vi "Engine.vi"() -> ()   [LabVIEW 2019]
uses:
  <vilib>/TaskbarProgressAPI/_TypeDefs/Progress State.ctl
  F:/src/Git/machine/CDL0100/TagEngine/LVOPCUA.NET/LVOPC.NETInterface/bin/Release/LVOPC.NETInterface.dll
  LVOPCUA.NET/LVOPC.NETInterface/bin/Release/LVOPC.NETInterface.dll
  <resource>/objmgr/ni.var.rc
  <vilib>/TaskbarProgressAPI/TaskbarProgressAPI.lvlib
panel:
  out "Scada Error":errorcluster
  out "Alarms SVE Size":i32
  out "Alarms Found":i32
  out "Listener ipAddr":string
  out "IP Addresses":string[](array[string])
  out "Basement Anybus OK":bool
  out "Profinet_Slaves_Connected":bool
  out "Profinet_Master_OK":bool
  out "Connected":i32
  out "Sweep Time":dbl(graph)
  out "Variables":i32
  out "Subscriptions":i32
  out "Sessions":i32
  out "Basement Rack Scanner":bool
  out "PLC Sweep Time":dbl
  out "PLC Sweep mode":string
  out "PLC Firmware":string
  out "PLC Date Code":string
  out "PLC Model":string
  out "error IO":errorcluster
  out "Loop Count":i32
  out "PSP Update Tm":dbl format="%#_4g"
  out "Wait Cycles":i32
  in  "stop":bool
  out "error out":errorcluster
  in  "PLC ipAddr":string="192.168.1.15"
  # "ms"
  # "OPC Server"
  # "Max=5"
  # "Max=10"
  # "Max=\n12,500"
  # "ms"
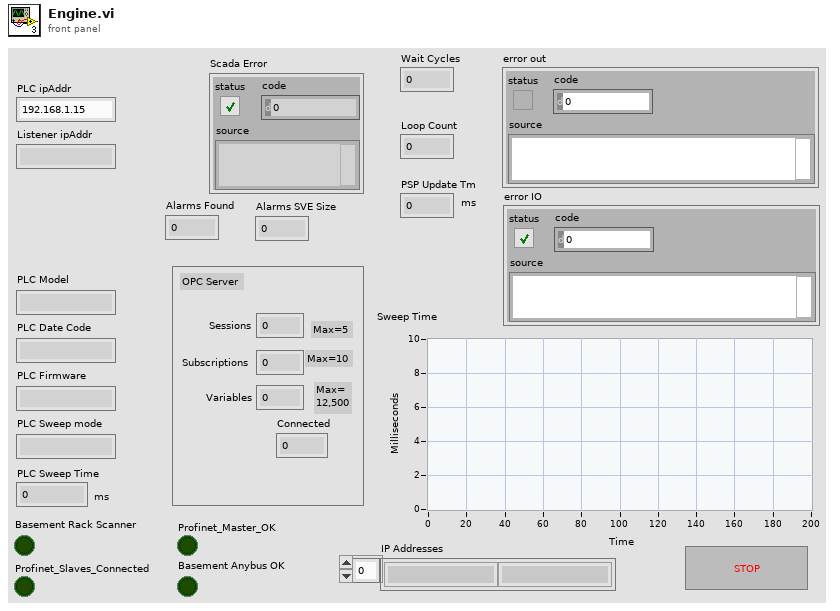
[diagram p1: front panel]
types:
  T1 = typedef "TaskbarProgressAPI.lvlib/Progress State.ctl" = i32
  T2 = typedef "Current Value Table.lvlib/Single Tag.ctl" = cluster{"Data Type":T3, "Name":string, "Value":string, "Description":string}
  T3 = typedef "Current Value Table.lvlib/Data Types.ctl" = enum16{"Double", "Single", "I64", "I32", "I16", "I8", "U64", "U32", "U16", "U8", "String", "Boolean", "Array of U8", "Array of U16", "Array of U32", "Array of U64", "Array of I64", "Array of I32", "Array of I16", "Array of I8", "Array of Double", "Array of Single", "Array of Boolean", "Array of String"}
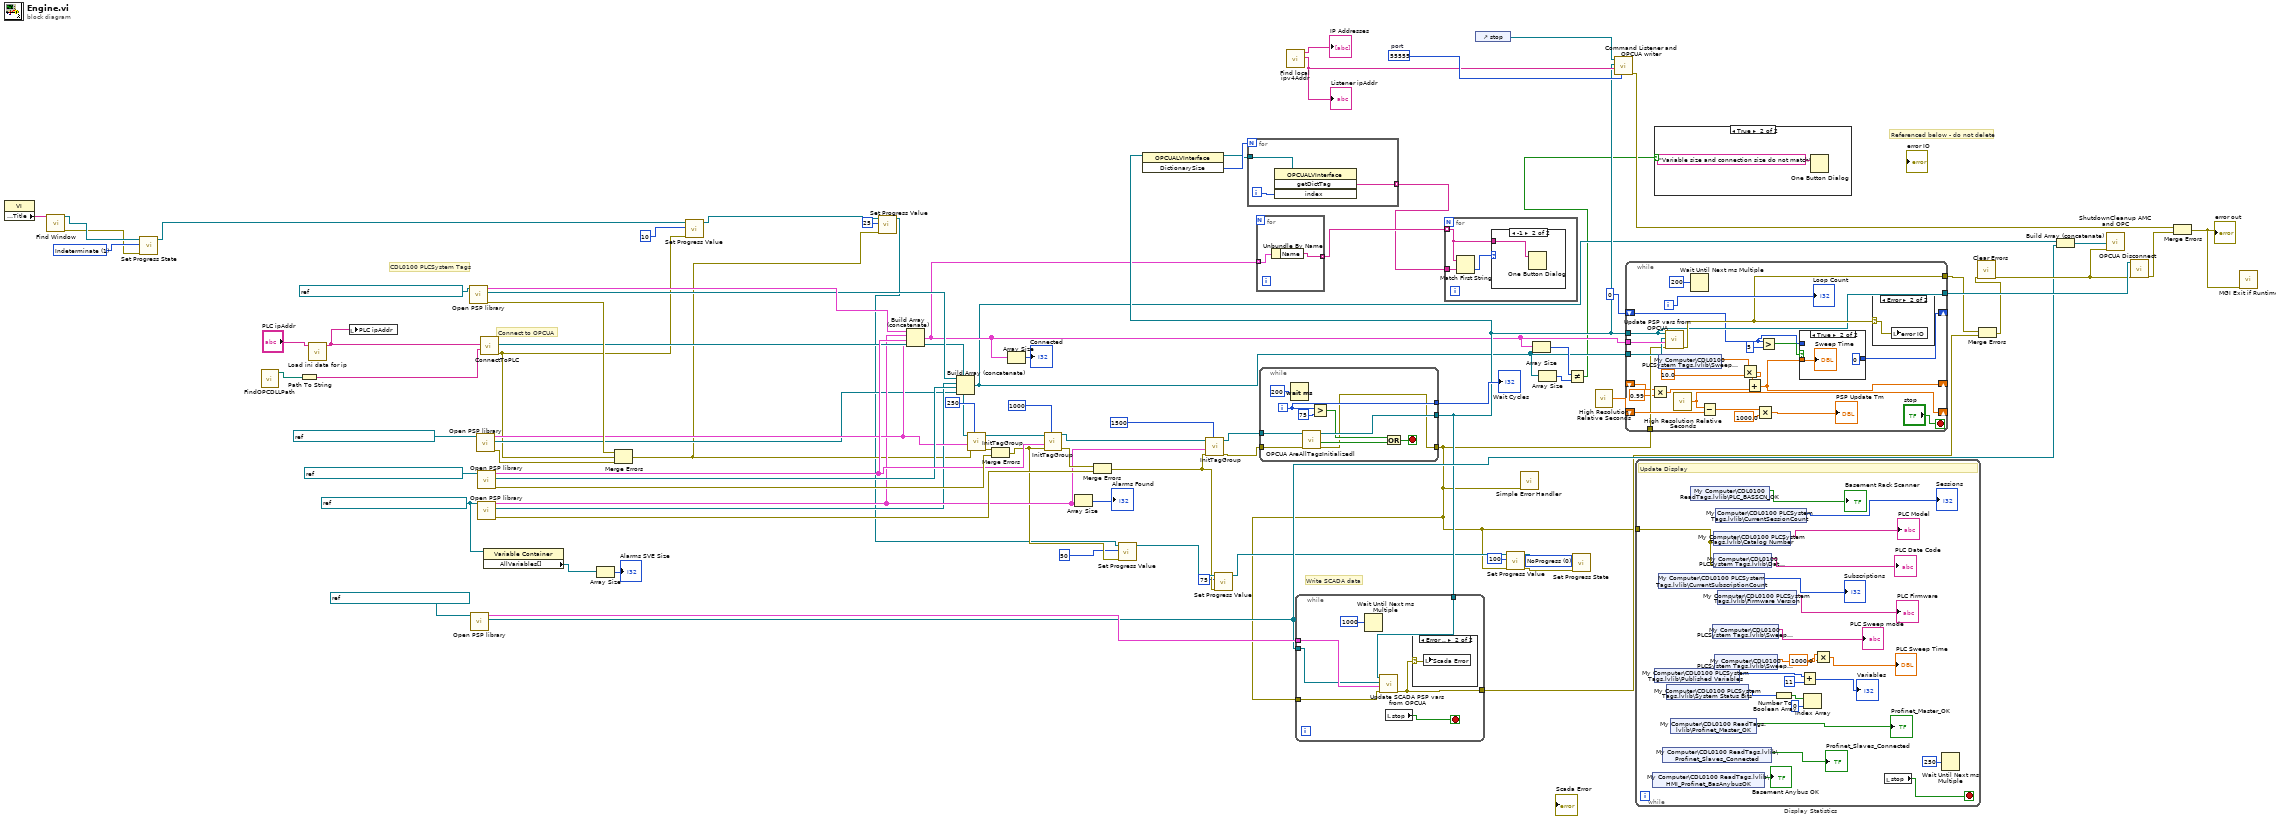
[diagram p0: block diagram]
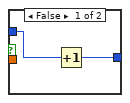
[diagram p5: hidden frame]
diagram:
  w1 = T1 0 items=["NoProgress"=0, "Indeterminate"=1, "Normal"=2, "Error"=4, "Paused"=8] ("State (No Progress)")
  w9 = T1 1 items=["NoProgress"=0, "Indeterminate"=1, "Normal"=2, "Error"=4, "Paused"=8] ("State (No Progress)")
  w45 = u16 55555  # port
  w36 = refnum<k21> "ni.var.psp://localhost/CDL0100 AlarmTags" ("container refnum in")
  # "Referenced below - do not delete"
  # "Write SCADA data"
  # "CDL0100 PLCSystem Tags"
  # "Connect to OPCUA"
  n1 = property class="VI"() -> ("Front Panel.Title"=w13:string)  [unwired: 2 in, 2 out]
  n2 = call <vilib>:"Find Window.vi"("Window Title (Callers Window)"=w13) -> ("error out"=w8:errorcluster, "Window Handle"=w11:refnum<k24>)  [unwired: 9 in]
  n3 = call <vilib>:"Set Progress State.vi"("error in (no error)"=w8, "State (No Progress)"=w9, "Window Handle"=w11) -> ("dup Window Handle"=w10:refnum<k24>)  [unwired: 7 in, 1 out]
  n4 = call "FindOPCDLLPath.vi"() -> ("DLL Path"=w66:path)  [unwired: 11 in]
  n5 = Path To String(path=w66) -> (string=w65:string)
  n6 = call "Load ini data for ip.vi"("PLC ipAddr"="PLC ipAddr") -> ("Selected IP addr"=w52:string)  [unwired: 10 in]
  n7 = local write "PLC ipAddr"(w52) -> ()
  n8 = call "Open PSP library.vi"("Refnum in"=refnum<k21> "ni.var.psp://localhost/CDL0100 PLCSystem Tags" ("container refnum in")) -> ("error out"=w76:errorcluster, "Variables"=w71:refnum<k21>[], "CVT Array"=w75:T2[])  [unwired: 8 in]
  n9 = call "Open PSP library.vi"("Refnum in"=refnum<k21> "ni.var.psp://huniopc01/CDL0100 SCADA") -> ("Variables"=w48:refnum<k21>[], "CVT Array"=w49:T2[])  [unwired: 8 in, 1 out]
  n10 = call "Open PSP library.vi"("Refnum in"=refnum<k21> "ni.var.psp://localhost/CDL0100 ReadTags" ("container refnum in")) -> ("error out"=w80:errorcluster, "Variables"=w30:refnum<k21>[], "CVT Array"=w33:T2[])  [unwired: 8 in]
  n11 = call "Open PSP library.vi"("Refnum in"=w36) -> ("error out"=w56:errorcluster, "Variables"=w31:refnum<k21>[], "CVT Array"=w32:T2[])  [unwired: 8 in]
  n12 = call "Open PSP library.vi"("Refnum in"=refnum<k21> "ni.var.psp://localhost/CDL0100 ReadWriteTags" ("container refnum in")) -> ("error out"=w82:errorcluster, "Variables"=w70:refnum<k21>[], "CVT Array"=w74:T2[])  [unwired: 8 in]
  n13 = call "ConnectToPLC.vi"("sDataDir"=w65, "ipAddr"=w52) -> ("error out"=w22:errorcluster, "Handle"=w69:refnum<k24>)  [unwired: 7 in, 1 out]
  n14 = property class="Variable Container"(reference=w36) -> ("AllVariables[]"=w35:refnum<k21>[])  [unwired: 1 in, 2 out]
  n15 = Array Size(array=w35) -> (size(s)=→"Alarms SVE Size":i32)
  n16 = Merge Errors(w76, w22, w80) -> (w21:errorcluster)
  n17 = call <vilib>:"Set Progress Value.vi"("error in (no error)"=w22, "current (0)"=10 ("Current Iteration"), "Window Handle"=w10) -> ("dup Window Handle"=w20:refnum<k24>)  [unwired: 7 in, 1 out]
  n18 = call <vilib>:"Set Progress Value.vi"("error in (no error)"=w21, "current (0)"=u64 25, "Window Handle"=w20) -> ("dup Window Handle"=w18:refnum<k24>)  [unwired: 7 in, 1 out]
  n19 = Build Array (concatenate)(w75, w32, w74, w33) -> (w29:T2[])
  n20 = Build Array (concatenate)(w71, w31, w70, w30) -> (w26:refnum<k21>[])
  n21 = call "InitTagGroup.vi"("updateInterval"=250, "error IO"=w21, "Tag List"=w33, "reference"=w69) -> ("error out"=w81:errorcluster, "reference 2"=w85:refnum<k24>)  [unwired: 4 in]
  n22 = Merge Errors(w81, w82) -> (w19:errorcluster)
  n23 = Array Size(array=w29) -> (size(s)=→"Connected":i32)
  n24 = call "InitTagGroup.vi"("updateInterval"=1000, "error IO"=w19, "Tag List"=w74, "reference"=w85) -> ("error out"=w57:errorcluster, "reference 2"=w58:refnum<k24>)  [unwired: 4 in]
  n25 = Array Size(array=w32) -> (size(s)=→"Alarms Found":i32)
  n26 = Merge Errors(w57, w56) -> (w16:errorcluster)
  n27 = call <vilib>:"Set Progress Value.vi"("error in (no error)"=w19, "current (0)"=u64 50, "Window Handle"=w18) -> ("dup Window Handle"=w17:refnum<k24>)  [unwired: 7 in, 1 out]
  n28 = call "InitTagGroup.vi"("updateInterval"=1500, "error IO"=w16, "Tag List"=w32, "reference"=w58) -> ("error out"=w23:errorcluster, "reference 2"=w55:refnum<k24>)  [unwired: 4 in]
  n29 = call <vilib>:"Set Progress Value.vi"("error in (no error)"=w16, "current (0)"=u64 75, "Window Handle"=w17) -> ("dup Window Handle"=w15:refnum<k24>)  [unwired: 7 in, 1 out]
  n30 = for {
    tunnel: w29 -> [w87] mode=indexing
    tunnel: [w86] -> w60 mode=indexing
    n31 = Unbundle By Name(w87) -> ("Name"=w86:string)
  }
  n32 = while {
    tunnel: w55 -> [w90]
    tunnel: w23 -> [w97]
    tunnel: [w96] -> w43
    tunnel: [w88] -> w14
    tunnel: [w89] -> w78
    i -> [w89]
    stop <- w92 stop-if-true
    n33 = Wait (ms)(milliseconds to wait=u32 200) -> ()  [unwired: 1 out]
    n34 = call "OPCUA AreAllTagsInitializedl.vi"("error in (no error)"=w97, "reference"=w90) -> ("error out"=w88:errorcluster, "Initialized"=w91:bool, "reference out"=w96:refnum<k24>)  [unwired: 7 in]
    n35 = Greater?(x=w89, y=75) -> (0:w93:bool)
    n36 = Or(x=w93, y=w91) -> (x .or. y?=w92:bool)
  }
  "Wait Cycles" <- w78
  n37 = invoke class="OPCUALVInterface" method="DictionarySize"(reference=w43) -> (reference out=w61:refnum<k24>, "DictionarySize"=w62:i32)  [unwired: 2 in, 1 out]
  n38 = for {
    N: w62 -> [_]
    tunnel: w61 -> [w100]
    tunnel: [w98] -> w59 mode=indexing
    i -> [w99]
    n39 = invoke class="OPCUALVInterface" method="getDictTag"(reference=w100, "index"=w99) -> ("getDictTag"=w98:string)  [unwired: 2 in, 3 out]
  }
  n40 = call "Find local ipv4Addr.vi"() -> ("name"=w44:string, "IP Addresses"=→"IP Addresses":string[])  [unwired: 10 in]
  "Listener ipAddr" <- w44
  n41 = while {
    tunnel: w48 -> [w103]
    tunnel: w49 -> [w104]
    tunnel: w43 -> [w105]
    tunnel: [w101] -> w40
    tunnel: w14 -> [w102]
    stop <- w106 stop-if-true
    n42 = Wait Until Next ms Multiple(millisecond multiple=u32 1000) -> ()  [unwired: 1 out]
    n43 = call "Update SCADA PSP vars from OPCUA.vi"("error in (no error)"=w102, "CVT Array"=w104, "Variables"=w103, "reference"=w105) -> ("error Out"=w101:errorcluster)  [unwired: 7 in]
    n44 = local read "stop"() -> (w106:bool)
    n45 = case shown="Error .." w101 {
      selector: w101 -> [_ w108]
      frame No Error {
      }
      frame Error {
        n46 = local write "Scada Error"(w108) -> ()
      }
    }
  }
  n47 = for {
    tunnel: w60 -> [w109] mode=indexing
    tunnel: w59 -> [w111]
    n48 = Match First String(2:w111, 3:w109) -> (0:w110:i32)  [unwired: 1 out]
    n49 = case shown="-1" w110 {
      tunnel: w109 -> [_ w112]
      frame 0, Default {
      }
      frame -1 {
        n50 = One Button Dialog(message=w112) -> ()  [unwired: 1 in, 1 out]
      }
    }
  }
  n51 = control-ref of="stop"() -> (w41:refnum<vi>)
  n52 = call <vilib>:"Set Progress Value.vi"("error in (no error)"=w14, "current (0)"=u64 100, "Window Handle"=w15) -> ("error out"=w2:errorcluster, "dup Window Handle"=w3:refnum<k24>)  [unwired: 7 in]
  n53 = call <vilib>:"Simple Error Handler.vi"("error in (no error)"=w14) -> ()  [unwired: 4 in, 5 out]
  n54 = Array Size(array=w29) -> (size(s)=w28:i32)
  n55 = Array Size(array=w26) -> (size(s)=w27:i32)
  n56 = Not Equal?(x=w28, y=w27) -> (x != y?=w25:bool)
  n57 = call <vilib>:"Set Progress State.vi"("error in (no error)"=w2, "State (No Progress)"=w1, "Window Handle"=w3) -> ()  [unwired: 7 in, 2 out]
  n58 = call <vilib>:"High Resolution Relative Seconds.vi"() -> ("relative seconds"=w77:dbl)
  n59 = call "Command Listener and OPCUA writer.vi"("port"=w45, "Server name"=w44, "OPCUA Connection in"=w43, "Stop Reference in"=w41) -> ("error out"=w42:errorcluster)  [unwired: 7 in]
  n60 = while {
    tunnel: w43 -> [w124]
    shift-right: [w134] -> _
    shift-left: w77 -> [w133]
    tunnel: w29 -> [w128]
    tunnel: w26 -> [w127]
    tunnel: w14 -> [w126]
    tunnel: [w125] -> w39
    tunnel: [w124] -> w68
    shift-right: [w117] -> _
    shift-left: _ -> [w121]
    shift-right: [w113] -> _
    shift-left: 0 -> [w114]
    i -> [w129]
    stop <- "stop" stop-if-true
    n61 = Multiply(x=w121, y=0.99) -> (x*y=w118:dbl)
    n62 = shared-variable "My Computer\\CDL0100 PLCSystem Tags.lvlib\\Sweep Time"() -> (w123:dbl)  [unwired: 1 in, 1 out]
    n63 = call "Update PSP vars from OPCUA.vi"("error in (no error)"=w126, "CVT Array"=w128, "Variables"=w127, "reference"=w124) -> ("error Out"=w125:errorcluster)  [unwired: 7 in]
    n64 = call <vilib>:"High Resolution Relative Seconds.vi"() -> ("relative seconds"=w134:dbl)
    n65 = Wait Until Next ms Multiple(millisecond multiple=u32 200) -> ()  [unwired: 1 out]
    n66 = Subtract(x=w134, y=w133) -> (x-y=w132:dbl)
    n67 = Multiply(x=w123, y=10.0) -> (x*y=w119:dbl)
    n68 = Add(x=w119, y=w118) -> (x+y=w117:dbl)
    n69 = Multiply(x=w132, y=1000.0) -> (x*y=→"PSP Update Tm":dbl)
    n70 = Greater?(x=w114, y=5) -> (0:w115:bool)
    n71 = case shown="True" w115 {
      tunnel: w117 -> [_ w140]
      tunnel: w114 -> [w138 _]
      tunnel: [w137 0] -> w113
      frame False {
        n72 = Increment(x=w138) -> (x+1=w137:i32)
      }
      frame True {
        "Sweep Time" <- w140
      }
    }
    n73 = case shown="Error" w125 {
      selector: w125 -> [_ w141]
      frame No Error {
      }
      frame Error {
        n74 = local write "error IO"(w141) -> ()
      }
    }
    "Loop Count" <- w129
  }
  n75 = while "Display Statistics" {
    tunnel: w14 -> [w160]
    stop <- w162 stop-if-true
    # "Update Display"
    n76 = shared-variable "My Computer\\CDL0100 ReadTags.lvlib\\HMI_Profinet_BasAnybusOK"() -> (→"Basement Anybus OK":bool)  [unwired: 1 in, 1 out]
    n77 = shared-variable "My Computer\\CDL0100 PLCSystem Tags.lvlib\\Published Variables"() -> (w144:i32)  [unwired: 1 in, 1 out]
    n78 = shared-variable "My Computer\\CDL0100 PLCSystem Tags.lvlib\\CurrentSubscriptionCount"() -> (→"Subscriptions":i32)  [unwired: 1 in, 1 out]
    n79 = shared-variable "My Computer\\CDL0100 ReadTags.lvlib\\Profinet_Slaves_Connected"() -> (→"Profinet_Slaves_Connected":bool)  [unwired: 1 in, 1 out]
    n80 = shared-variable "My Computer\\CDL0100 PLCSystem Tags.lvlib\\System Status Bits"() -> (w157:i32)  [unwired: 1 in, 1 out]
    n81 = shared-variable "My Computer\\CDL0100 ReadTags.lvlib\\Profinet_Master_OK"() -> (→"Profinet_Master_OK":bool)  [unwired: 1 in, 1 out]
    n82 = shared-variable "My Computer\\CDL0100 ReadTags.lvlib\\PLC_BASSCN_OK"() -> (→"Basement Rack Scanner":bool)  [unwired: 1 in, 1 out]
    n83 = shared-variable "My Computer\\CDL0100 PLCSystem Tags.lvlib\\Sweep Mode"() -> (→"PLC Sweep mode":string)  [unwired: 1 in, 1 out]
    n84 = shared-variable "My Computer\\CDL0100 PLCSystem Tags.lvlib\\Catalog Number"(error in=w160) -> (→"PLC Model":string)  [unwired: 1 out]
    n85 = shared-variable "My Computer\\CDL0100 PLCSystem Tags.lvlib\\Date Code"(error in=w160) -> (→"PLC Date Code":string)  [unwired: 1 out]
    n86 = shared-variable "My Computer\\CDL0100 PLCSystem Tags.lvlib\\Sweep Time"() -> (w147:dbl)  [unwired: 1 in, 1 out]
    n87 = shared-variable "My Computer\\CDL0100 PLCSystem Tags.lvlib\\CurrentSessionCount"() -> (→"Sessions":i32)  [unwired: 1 in, 1 out]
    n88 = shared-variable "My Computer\\CDL0100 PLCSystem Tags.lvlib\\Firmware Version"() -> (→"PLC Firmware":string)  [unwired: 1 in, 1 out]
    n89 = Number To Boolean Array(number=w157) -> (Boolean array=w156:bool[])
    n90 = Add(x=w144, y=11) -> (x+y=→"Variables":i32)
    n91 = Index Array(array=w156, index=0) -> ()  [unwired: 1 out]
    n92 = Multiply(x=w147, y=1000.0) -> (x*y=→"PLC Sweep Time":dbl)
    n93 = local read "stop"() -> (w162:bool)
    n94 = Wait Until Next ms Multiple(millisecond multiple=u32 250) -> ()  [unwired: 1 out]
  }
  n95 = case shown="True" w25 {
    frame False {
    }
    frame True {
      n96 = One Button Dialog(message="Variable size and connection size do not match") -> ()  [unwired: 1 in, 1 out]
    }
  }
  n97 = Merge Errors(w39, w40) -> (w38:errorcluster)
  n98 = call <vilib>:"Clear Errors.vi"("error in (no error)"=w38) -> ("error out"=w67:errorcluster)  [unwired: 5 in, 1 out]
  n99 = Build Array (concatenate)(w26, w48) -> (w47:refnum<k21>[])
  n100 = call "ShutdownCleanup AMC and OPC.vi"("error in (no error)"=w67, "Array of Variables"=w47) -> ()  [unwired: 10 in]
  n101 = call "OPCUA Disconnect.vi"("error in (no error)"=w67, "reference"=w68) -> ("error out"=w64:errorcluster)  [unwired: 8 in, 1 out]
  n102 = Merge Errors(w42, w64) -> (w24:errorcluster)
  "error out" <- w24
  n103 = call <userlib>:"MGI Exit if Runtime.vi"("Error In (Dependency Only)"=w24) -> ()  [unwired: 11 in]
